vi "magic PSP open.vi"(7 "var string in":string[](array[string]), 8 "error in (no error)":errorcluster, 10 "timeout (ms)":u32=1000, 11 "vars in":refnum<k21>[](array[refnum])) -> (0 "error out":errorcluster, 2 "Times (ms)":dbl[](array[numeric]), 3 "Vars out":refnum<k21>[](array[refnum]))   [LabVIEW 2026, in "TALOS.lvlib" / "Classes.lvlib" / "Circus Shared Variables.lvclass"]
uses:
  Circus Shared Variables.lvclass
  <resource>/objmgr/ni.var.rc
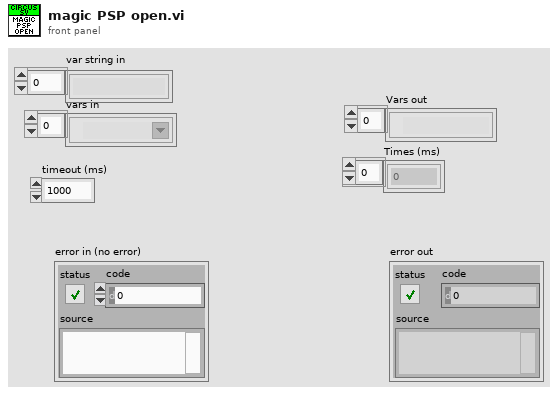
[diagram p1: front panel]
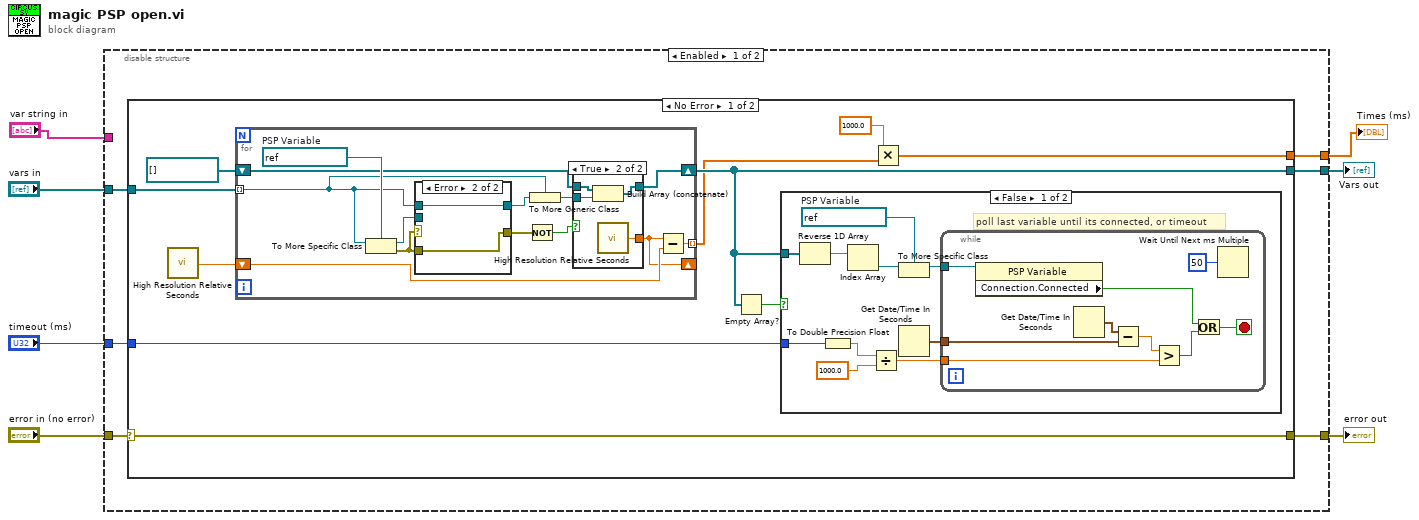
[diagram p0: block diagram]
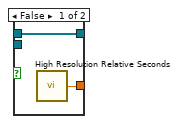
[diagram p2: hidden frame]
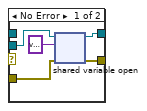
[diagram p3: hidden frame]
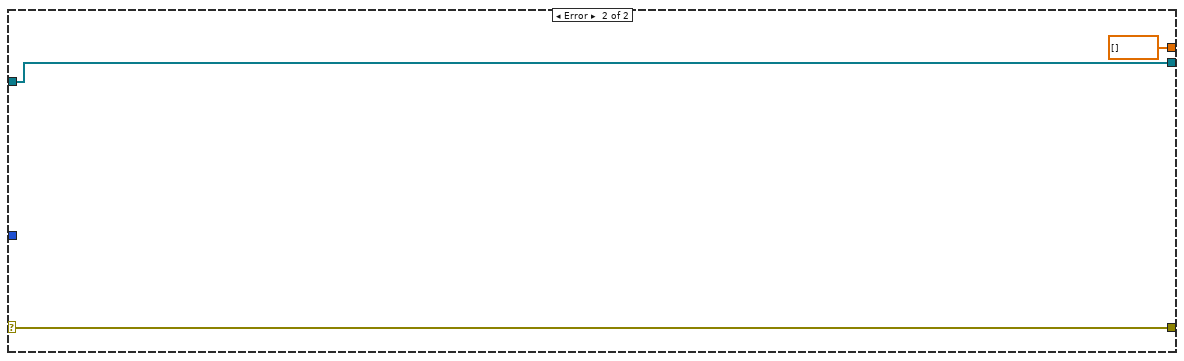
[diagram p5: hidden frame]
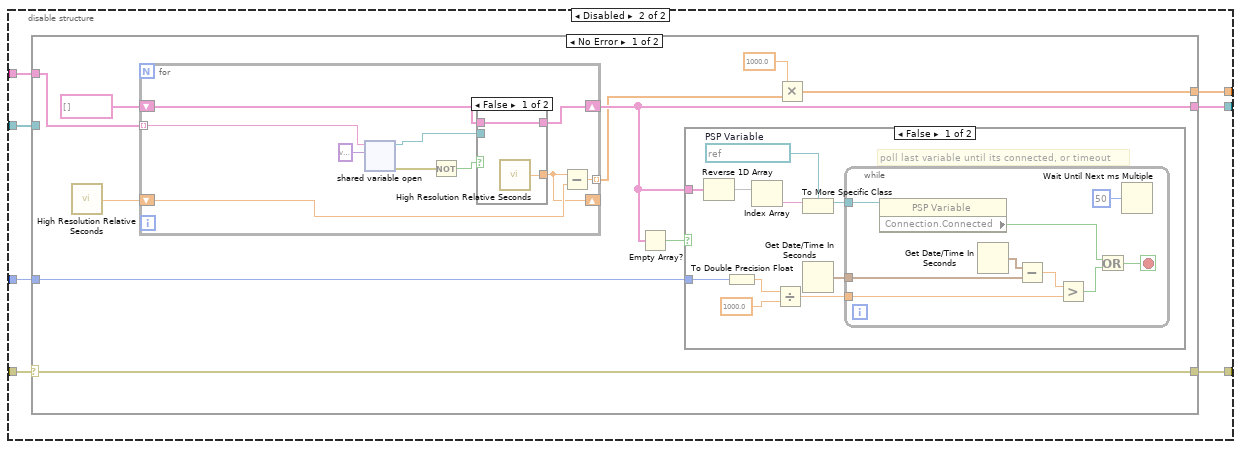
[diagram p6: hidden frame]
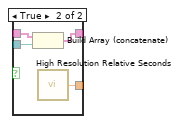
[diagram p7: hidden frame]
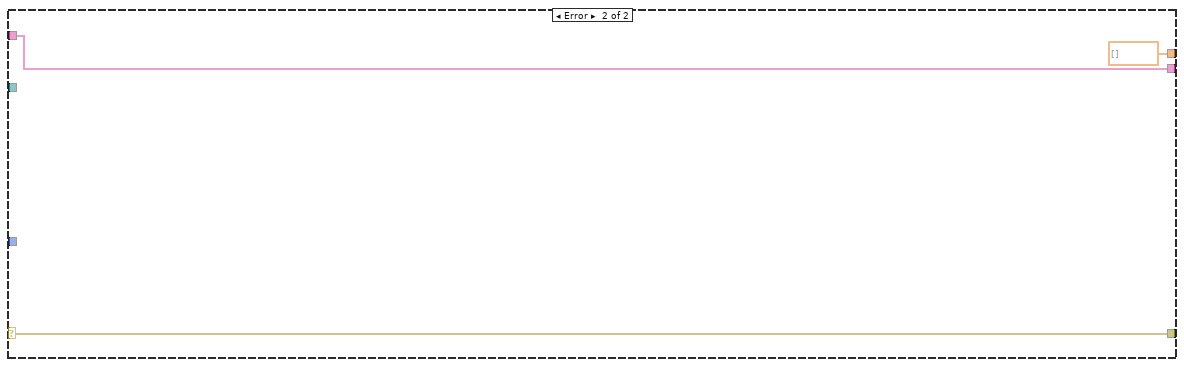
[diagram p9: hidden frame]
diagram:
  n1 = disable-structure shown="Enabled" {
    disable-tunnel: "vars in" -> [w13 w78]
    disable-tunnel: [w12 w73] -> w6
    disable-tunnel: "timeout (ms)" -> [w11 w77]
    disable-tunnel: "error in (no error)" -> [w10 w76]
    disable-tunnel: [w9 w75] -> w3
    disable-tunnel: "var string in" -> [_ w74]
    disable-tunnel: [w8 w72] -> w1
    frame Enabled {
      n2 = case shown="No Error" w10 {
        selector: w10 -> [w18 w71]
        tunnel: w13 -> [w23 w70]
        tunnel: [w22 w70] -> w12
        tunnel: w11 -> [w20 _]
        tunnel: [w18 w71] -> w9
        tunnel: [w14 dbl[] []] -> w8
        frame No Error {
          n3 = call <vilib>:"High Resolution Relative Seconds.vi"() -> ("relative seconds"=w17:dbl)
          n4 = for {
            tunnel: w23 -> [w29] mode=indexing
            shift-right: [w27] -> w22
            shift-left: refnum<k21>[] [] ("Array") -> [w28]
            tunnel: [w26] -> w15 mode=indexing
            shift-right: [w24] -> _
            shift-left: w17 -> [w25]
            w36 = refnum<k21> refnum  # PSP Variable
            n5 = To More Specific Class(target class=w36, reference=w29) -> (specific class reference=w35:refnum<k21>, error out=w31:errorcluster)  [unwired: 1 in]
            n6 = case shown="Error" w31 {
              tunnel: w35 -> [w47 _]
              tunnel: w31 -> [w46 w48]
              tunnel: [w45 w49] -> w34
              tunnel: [w44 w48] -> w32
              tunnel: w29 -> [_ w49]
              frame No Error {
                n7 = shared-variable-open(w47, w46, variant ("data")) -> (w45:refnum<k21>, w44:errorcluster)  [unwired: 2 in]
              }
              frame Error {
              }
            }
            n8 = Not(x=w32) -> (.not. x?=w33:bool)
            n9 = To More Generic Class(target class=w29, reference=w34) -> (generic class reference=w30:refnum<k21>)
            n10 = case shown="True" w33 {
              tunnel: w28 -> [w38 w41]
              tunnel: w30 -> [_ w40]
              tunnel: [w38 w42] -> w27
              tunnel: [w37 w39] -> w24
              frame False {
                n11 = call <vilib>:"High Resolution Relative Seconds.vi"() -> ("relative seconds"=w37:dbl)
              }
              frame True {
                n12 = Build Array (concatenate)(w41, w40) -> (w42:refnum<k21>[])
                n13 = call <vilib>:"High Resolution Relative Seconds.vi"() -> ("relative seconds"=w39:dbl)
              }
            }
            n14 = Subtract(x=w24, y=w25) -> (x-y=w26:dbl)
          }
          n15 = Empty Array?(array=w22) -> (empty?=w21:bool)
          n16 = case shown="False" w21 {
            tunnel: w22 -> [w58 _]
            tunnel: w20 -> [w52 _]
            frame False {
              w57 = refnum<k21> refnum  # PSP Variable
              # "poll last variable until its connected, or timeout"
              n17 = Reverse 1D Array(array=w58) -> (reversed array=w59:refnum<k21>[])
              n18 = To Double Precision Float(number=w52) -> (double precision float=w51:dbl)
              n19 = Index Array(array=w59) -> (element=w56:refnum<k21>)  [unwired: 1 in]
              n20 = Divide(x=w51, y=1000.0) -> (x/y=w53:dbl)
              n21 = To More Specific Class(target class=w57, reference=w56) -> (specific class reference=w55:refnum<k21>)  [unwired: 1 in, 1 out]
              n22 = Get Date/Time In Seconds() -> (seconds since 1Jan1904=w54:timestamp)
              n23 = while {
                tunnel: w55 -> [w68]
                tunnel: w54 -> [w65]
                tunnel: w53 -> [w60]
                stop <- w63 stop-if-true
                n24 = property class="PSP Variable"(reference=w68) -> ("Connection.Connected"=w67:bool)  [unwired: 1 in, 2 out]
                n25 = Get Date/Time In Seconds() -> (seconds since 1Jan1904=w66:timestamp)
                n26 = Subtract(x=w66, y=w65) -> (x-y=w64:dbl)
                n27 = Greater?(x=w64, y=w60) -> (0:w62:bool)
                n28 = Or(x=w67, y=w62) -> (x .or. y?=w63:bool)
                n29 = Wait Until Next ms Multiple(millisecond multiple=u32 50) -> ()  [unwired: 1 out]
              }
            }
            frame True {
            }
          }
          n30 = Multiply(x=1000.0, y=w15) -> (x*y=w14:dbl[])
        }
        frame Error {
        }
      }
    }
    frame Disabled {
      n31 = case shown="No Error" w76 {
        selector: w76 -> [w84 w126]
        tunnel: w78 -> [_ _]
        tunnel: [w88 w125] -> w73
        tunnel: w77 -> [w86 _]
        tunnel: [w84 w126] -> w75
        tunnel: w74 -> [w80 w125]
        tunnel: [w79 dbl[] []] -> w72
        frame No Error {
          n32 = call <vilib>:"High Resolution Relative Seconds.vi"() -> ("relative seconds"=w83:dbl)
          n33 = for {
            tunnel: w80 -> [w89] mode=indexing
            shift-right: [w95] -> w88
            shift-left: string[] [] ("Array") -> [w96]
            tunnel: [w94] -> w81 mode=indexing
            shift-right: [w92] -> _
            shift-left: w83 -> [w93]
            n34 = shared-variable-open(w89, variant ("data")) -> (w91:refnum<k21>, w97:errorcluster)  [unwired: 3 in]
            n35 = Not(x=w97) -> (.not. x?=w98:bool)
            n36 = case shown="False" w98 {
              tunnel: w96 -> [w100 w103]
              tunnel: w91 -> [_ w102]
              tunnel: [w100 w104] -> w95
              tunnel: [w99 w101] -> w92
              frame False {
                n37 = call <vilib>:"High Resolution Relative Seconds.vi"() -> ("relative seconds"=w99:dbl)
              }
              frame True {
                n38 = Build Array (concatenate)(w103, w102) -> (w104:string[])
                n39 = call <vilib>:"High Resolution Relative Seconds.vi"() -> ("relative seconds"=w101:dbl)
              }
            }
            n40 = Subtract(x=w92, y=w93) -> (x-y=w94:dbl)
          }
          n41 = Empty Array?(array=w88) -> (empty?=w87:bool)
          n42 = case shown="False" w87 {
            tunnel: w88 -> [w113 _]
            tunnel: w86 -> [w107 _]
            frame False {
              w112 = refnum<k21> refnum  # PSP Variable
              # "poll last variable until its connected, or timeout"
              n43 = Reverse 1D Array(array=w113) -> (reversed array=w114:string[])
              n44 = To Double Precision Float(number=w107) -> (double precision float=w106:dbl)
              n45 = Index Array(array=w114) -> (element=w111:string)  [unwired: 1 in]
              n46 = Divide(x=w106, y=1000.0) -> (x/y=w108:dbl)
              n47 = To More Specific Class(target class=w112, reference=w111) -> (specific class reference=w110:refnum<k21>)  [unwired: 1 in, 1 out]
              n48 = Get Date/Time In Seconds() -> (seconds since 1Jan1904=w109:timestamp)
              n49 = while {
                tunnel: w110 -> [w123]
                tunnel: w109 -> [w120]
                tunnel: w108 -> [w115]
                stop <- w118 stop-if-true
                n50 = property class="PSP Variable"(reference=w123) -> ("Connection.Connected"=w122:bool)  [unwired: 1 in, 2 out]
                n51 = Get Date/Time In Seconds() -> (seconds since 1Jan1904=w121:timestamp)
                n52 = Subtract(x=w121, y=w120) -> (x-y=w119:dbl)
                n53 = Greater?(x=w119, y=w115) -> (0:w117:bool)
                n54 = Or(x=w122, y=w117) -> (x .or. y?=w118:bool)
                n55 = Wait Until Next ms Multiple(millisecond multiple=u32 50) -> ()  [unwired: 1 out]
              }
            }
            frame True {
            }
          }
          n56 = Multiply(x=1000.0, y=w81) -> (x*y=w79:dbl[])
        }
        frame Error {
        }
      }
    }
  }
  "Vars out" <- w6
  "error out" <- w3
  "Times (ms)" <- w1
